vi "GOOP_ClassTemplateSplit.vi"(2 "ClassItemRefIn":refnum<vi>, 5 "FullClassTemplate":string) -> (4 "StandardTemplate":string, 8 "AF Template":string)   [LabVIEW 2020, in "ClassWriterNative.lvclass"]
uses:
  ClassProviders/Provider_LvNativeClass/ClassWriterNative_class/ClassWriterNative.lvclass
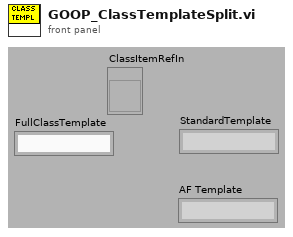
[diagram p1: front panel]
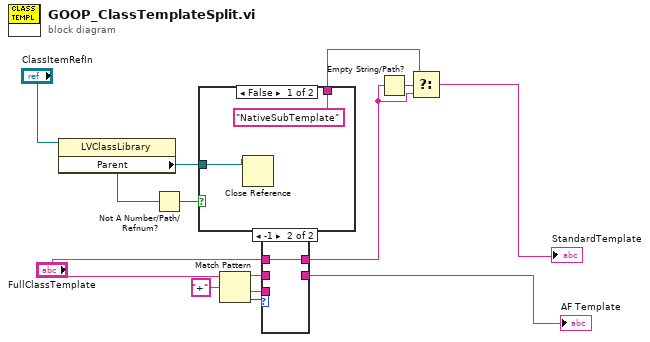
[diagram p0: block diagram]
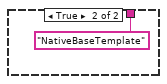
[diagram p2: hidden frame]
diagram:
  n1 = property class="LVClassLibrary"(reference="ClassItemRefIn") -> ("Parent"=w3:refnum<vi>)  [unwired: 1 in, 2 out]
  n2 = Not A Number/Path/Refnum?(number/path/refnum=w3) -> (NaN/Path/Refnum?=w4:bool)
  n3 = case shown="False" w4 {
    tunnel: ["NativeSubTemplate" ("t") "NativeBaseTemplate" ("t")] -> w6
    tunnel: w3 -> [w14 _]
    frame False {
      n4 = Close Reference(reference=w14) -> ()  [unwired: 1 in, 1 out]
    }
    frame True {
    }
  }
  n5 = Match Pattern(string="FullClassTemplate", regular expression="+") -> (before substring=w9:string, after substring=w13:string, offset past match=w11:i32)  [unwired: 1 in, 1 out]
  n6 = case shown="-1" w11 {
    tunnel: "FullClassTemplate" -> [_ w19]
    tunnel: [w18 w19] -> w2
    tunnel: w13 -> [w18 _]
    tunnel: [w17 _] -> w8
    tunnel: w9 -> [w17 _]
    frame 0, Default {
    }
    frame -1 {
    }
  }
  "AF Template" <- w8
  n7 = Empty String/Path?(string/path=w2) -> (empty?=w7:bool)
  n8 = Select(t=w6, s=w7, f=w2) -> (s? t:f=→"StandardTemplate":string)
